vi "paramrangemaker.vi"(11 "peakrangedata":T2) -> (3 "parameter bounds out":T1)   [LabVIEW 2020]
panel:
  out "parameter bounds":T1
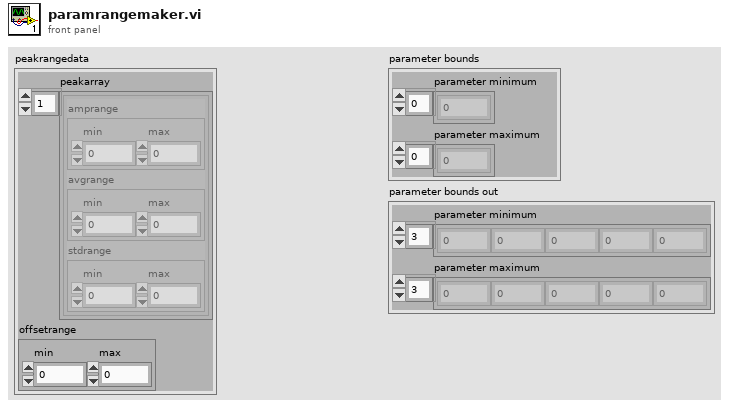
[diagram p1: front panel]
types:
  T1 = cluster{"parameter minimum":dbl[], "parameter maximum":dbl[]}
  T2 = cluster{"peakarray":cluster{"amprange":cluster{"min":dbl, "max":dbl}, "avgrange":cluster{"min":dbl, "max":dbl}, "stdrange":cluster{"min":dbl, "max":dbl}}[], "offsetrange":cluster{"min":dbl, "max":dbl}}
  T3 = cluster{"amprange":cluster{"min":dbl, "max":dbl}, "avgrange":cluster{"min":dbl, "max":dbl}, "stdrange":cluster{"min":dbl, "max":dbl}}[]
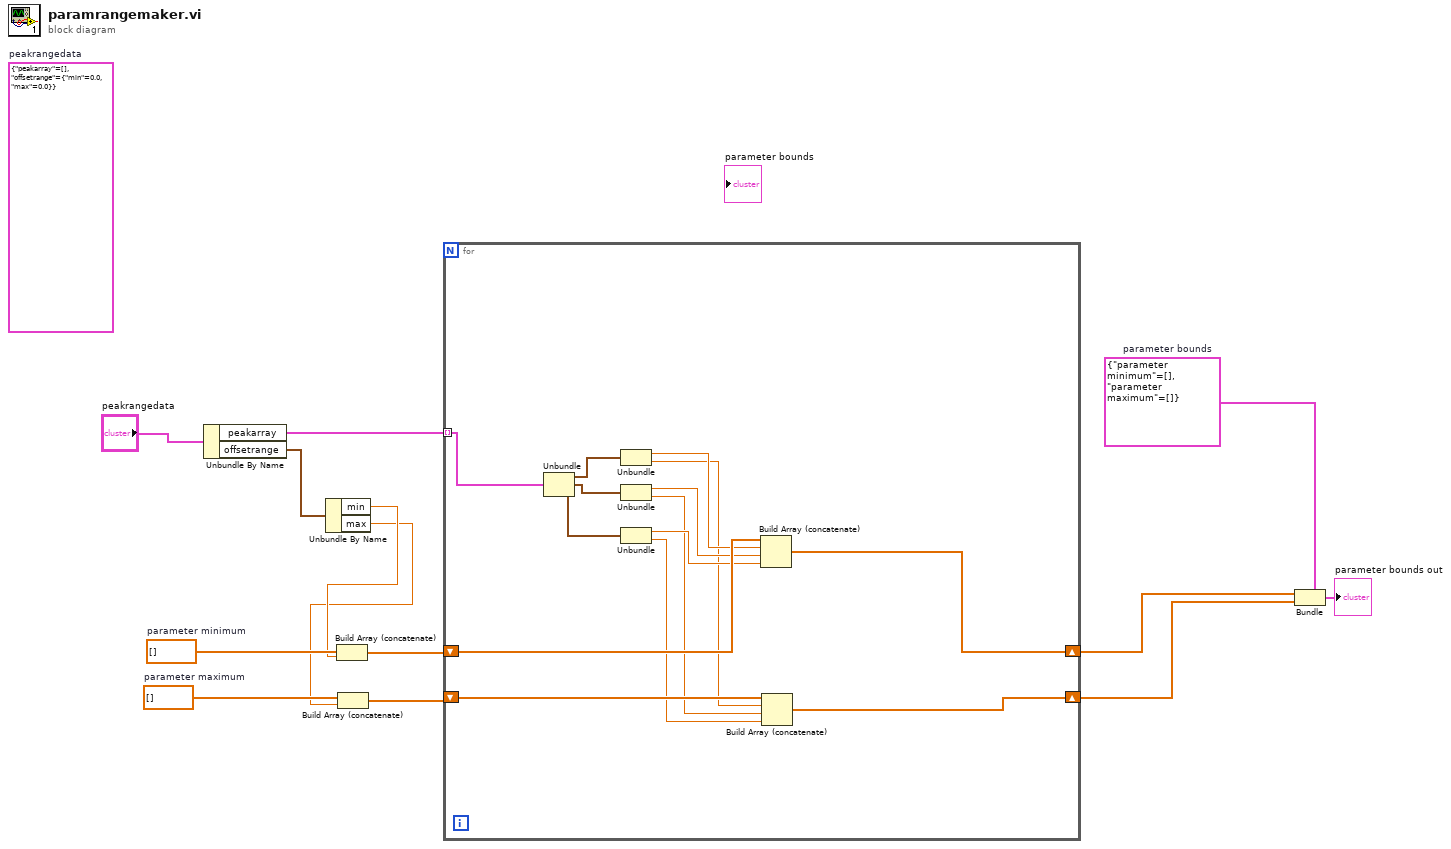
[diagram p0: block diagram]
diagram:
  w9 = dbl[] []  # parameter maximum
  w11 = dbl[] []  # parameter minimum
  w4 = T1 {"parameter minimum"=[], "parameter maximum"=[]}  # parameter bounds
  (unwired) T2 {"peakarray"=[], "offsetrange"={"min"=0.0, "max"=0.0}}  # peakrangedata
  n1 = Unbundle By Name("peakrangedata") -> ("peakarray"=w12:T3, "offsetrange"=w7:cluster{"min":dbl, "max":dbl})
  n2 = Unbundle By Name(w7) -> ("min"=w6:dbl, "max"=w5:dbl)
  n3 = Build Array (concatenate)(w11, w6) -> (w10:dbl[])
  n4 = Build Array (concatenate)(w9, w5) -> (w8:dbl[])
  n5 = for {
    tunnel: w12 -> [w27] mode=indexing
    shift-right: [w15] -> w3
    shift-left: w10 -> [w25]
    shift-right: [w14] -> w2
    shift-left: w8 -> [w24]
    n6 = Unbundle(w27) -> ("amprange"=w26:cluster{"min":dbl, "max":dbl}, "avgrange"=w23:cluster{"min":dbl, "max":dbl}, "stdrange"=w22:cluster{"min":dbl, "max":dbl})
    n7 = Unbundle(w26) -> ("min"=w21:dbl, "max"=w18:dbl)
    n8 = Unbundle(w23) -> ("min"=w20:dbl, "max"=w17:dbl)
    n9 = Unbundle(w22) -> ("min"=w19:dbl, "max"=w16:dbl)
    n10 = Build Array (concatenate)(w25, w21, w20, w19) -> (w15:dbl[])
    n11 = Build Array (concatenate)(w24, w18, w17, w16) -> (w14:dbl[])
  }
  n12 = Bundle(cluster=w4, "parameter minimum"=w3, "parameter maximum"=w2) -> (→"parameter bounds out":T1)
